vi "DVR Buffer.vi"(8 "error in (no error)":errorcluster) -> (0 "error out":errorcluster, 3 "DVR Out":refnum<data-value>)   [LabVIEW 2015]
uses:
  Systype.ctl
  Message Queue/Message Cluster.ctl
  Message Queue/Message Queue.lvlib
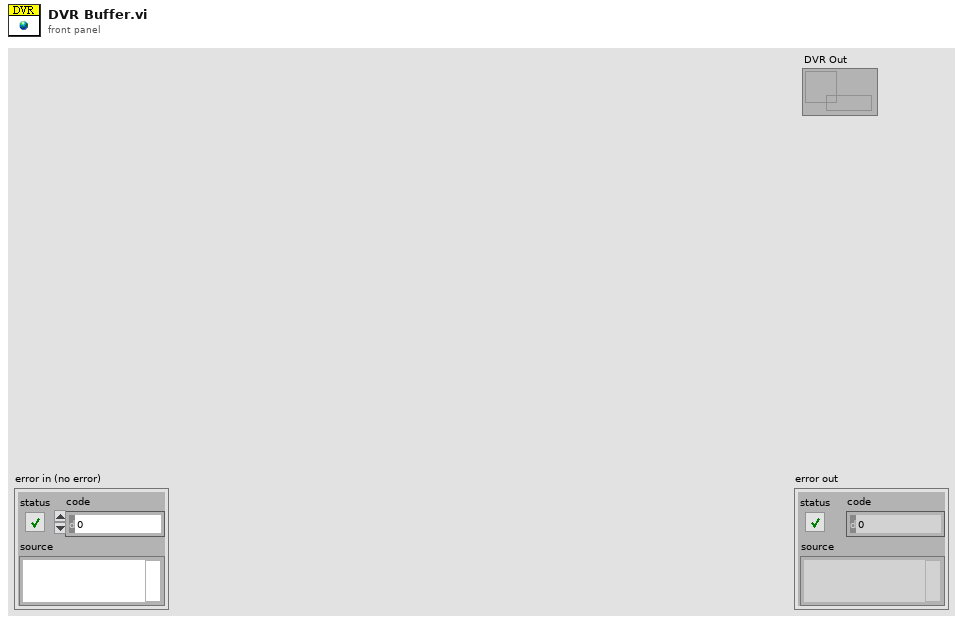
[diagram p1: front panel]
types:
  T1 = typedef "Systype.ctl" = cluster{"Message":cluster{"UI":refnum<queue>, "Task":refnum<queue>}, "VIParameter":cluster{"UI Ctrls":cluster{"Ctl Refnum":refnum<vi>}, "VIPath":path, "DataPath":path, "Project":string, "VIRef":refnum<vi>, "Stop":refnum<user-event>}, "InspectParameter":cluster{"Top":cluster{"ROI Descriptor":T2}}}
  T2 = typedef "ROI Descriptor" = cluster{"Global Rectangle":i32[], "Contours":cluster{"ID":enum32{"External", "Internal"}, "Type":u32, "Coordinates":i32[]}[]}
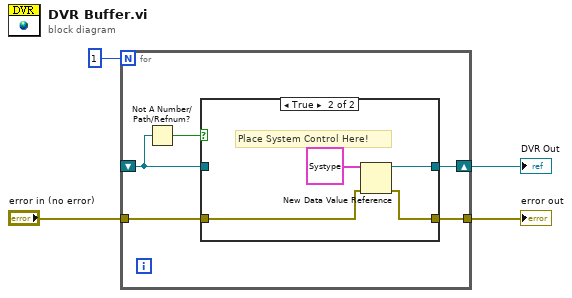
[diagram p0: block diagram]
diagram:
  n1 = for {
    N: 1 -> [_]
    shift-right: [w6] -> w1
    shift-left: _ -> [w8]
    tunnel: "error in (no error)" -> [w7]
    tunnel: [w5] -> w2
    n2 = Not A Number/Path/Refnum?(number/path/refnum=w8) -> (NaN/Path/Refnum?=w9:bool)
    n3 = case shown="True" w9 {
      tunnel: [w11 w15] -> w6
      tunnel: w8 -> [w11 _]
      tunnel: [w10 w14] -> w5
      tunnel: w7 -> [w10 w13]
      frame False {
      }
      frame True {
        # "Place System Control Here!"
        n4 = New Data Value Reference(data value=T1 {"Message"={"UI"=refnum, "Task"=refnum}, "VIParameter"={"UI Ctrls"={"Ctl Refnum"=refnum}, "VIPath"=path "", "DataPath"=path "", "Project"="", "VIRef"=refnum, "Stop"=refnum}, "InspectParameter"={"Top"={"ROI Descriptor"={"Global Rectangle"=[], "Contours"=[]}}}} ("SysType"), error in=w13) -> (data value reference=w15:refnum<data-value>, error out=w14:errorcluster)
      }
    }
  }
  "error out" <- w2
  "DVR Out" <- w1
